vi "Producto Seleccionado.vi"(8 "error in (no error)":errorcluster, 10 "Multicolumn Productos":i32(listbox), 11 "CAFE ACTOR in":refnum<class "CAFE ACTOR.lvclass">) -> (0 "error out":errorcluster, 3 "CAFE ACTOR out":refnum<class "CAFE ACTOR.lvclass">)   [LabVIEW 2019, in "CAFE ACTOR.lvlib" / "CAFE ACTOR.lvclass"]
uses:
  CAFE ACTOR.lvclass
  C:/Program Files (x86)/National Instruments/LabVIEW 2019/vi.lib/ActorFramework/Actor/Actor.lvclass
  <vilib>/ActorFramework/Actor/Actor.lvclass/Actor.ctl
  CAFE ACTOR.lvclass/CAFE ACTOR.ctl
  UI Actor Messages/Producto Seleccionado Msg/Producto Seleccionado Msg.lvclass/Producto Seleccionado Msg.ctl
  <vilib>/ActorFramework/Message Enqueuer/Message Enqueuer.lvclass/Message Enqueuer.ctl
  <vilib>/ActorFramework/Message Enqueuer/Enqueue.vi
  UI Actor Messages/Producto Seleccionado Msg/Producto Seleccionado Msg.lvclass
  C:/Program Files (x86)/National Instruments/LabVIEW 2019/vi.lib/ActorFramework/Message/Message.lvclass
  <vilib>/ActorFramework/Message Priority Queue/Priority Enqueue.vi
  <vilib>/ActorFramework/Actor/Actor.lvclass
panel:
  in  "array":string[](array[string])
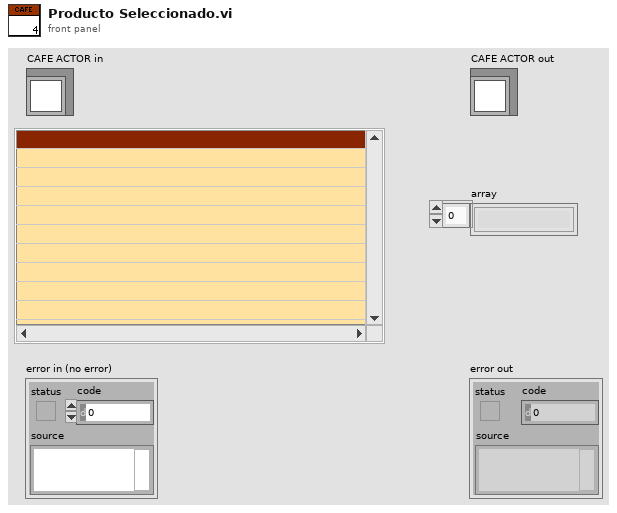
[diagram p1: front panel]
types:
  T1 = cluster{"array[0]":string, "array[1]":string, "array[2]":string, "array[3]":string, "array[4]":string, "array[5]":string, "array[6]":string, "array[7]":string, "array[8]":string}
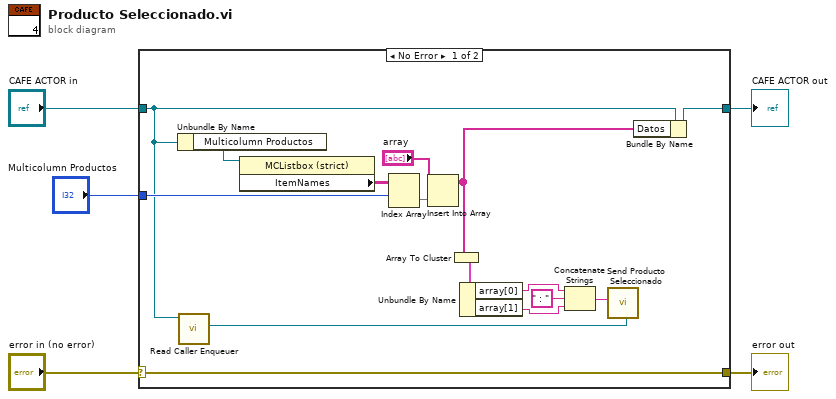
[diagram p0: block diagram]
diagram:
  n1 = case shown="No Error" "error in (no error)" {
    selector: "error in (no error)" -> [w20 w22]
    tunnel: [w20 w22] -> w2
    tunnel: [w10 w21] -> w5
    tunnel: "CAFE ACTOR in" -> [w8 w21]
    tunnel: "Multicolumn Productos" -> [w11 _]
    frame No Error {
      n2 = Unbundle By Name(w8) -> ("Multicolumn Productos"=w9:refnum<vi>)
      n3 = call <vilib>:"Read Caller Enqueuer.vi"("Actor"=w8) -> ("Caller Enqueuer"=w7:refnum<class "Message Enqueuer.lvclass">)  [unwired: 10 in]
      n4 = property on="Property Node" class="MCListbox (strict)"(reference=w9) -> ("ItemNames"=w17:string[][])  [unwired: 1 in, 2 out]
      n5 = Index Array(array=w17, index (row)=w11) -> (element=w18:string[])  [unwired: 1 in]
      n6 = Insert Into Array(array="array", new element=w18) -> (w12:string[])  [unwired: 1 in]
      n7 = Array To Cluster(array=w12) -> (cluster=w13:T1)
      n8 = Unbundle By Name(w13) -> ("array[0]"=w15:string, "array[1]"=w14:string)
      n9 = Concatenate Strings(w15, " : " ("string"), w14) -> (w6:string)
      n10 = call "Send Producto Seleccionado.vi"("Producto Seleccionado"=w6, "Message Enqueuer"=w7) -> ()  [unwired: 8 in, 2 out]
      n11 = Bundle By Name(cluster=w8, "Datos"=w12) -> (w10:refnum<class "CAFE ACTOR.lvclass">)
    }
    frame Error {
    }
  }
  "error out" <- w2
  "CAFE ACTOR out" <- w5
